vi "Create Evaluations.vi"(8 "error in (no error)":errorcluster, 11 "SPECAN_PVT in":refnum<class "SPECAN_PVT.lvclass">) -> (0 "error out":errorcluster, 1 "Evaluations Out":T1[](array[typedef]) {"Low Limit" format="%#_13g"; "SI Scaling" items=["femto"=-15, "pico"=-12, "nano"=-9, "micro"=-6, "milli"=-3, "percent"=-2, ""=0, "kilo"=3, "mega"=6, "giga"=9, "tera"=12]}, 3 "SPECAN_PVT out":refnum<class "SPECAN_PVT.lvclass">)   [LabVIEW 2018, in "SPECAN_PVT.lvlib" / "SPECAN_PVT.lvclass"]
uses:
  SPECAN_PVT.lvclass
  Plugins/TestStand API Tools (TSAT).lvlibp/Evaluation Actions/Includes/Controls/TSAT Evaluation.ctl
  Plugins/TestStand API Tools (TSAT).lvlibp/Evaluation Actions/Includes/Controls/TSAT Eval SI Unit Scaling.ctl
  Plugins/TestStand API Tools (TSAT).lvlibp/Evaluation Actions/Includes/Controls/TSAT Evaluation Type.ctl
  SPECAN_PVT.lvclass/SPECAN_PVT.ctl
  Plugins/SeqAuto Evaluations.lvlibp/ModeSwitch/ModeSwitch Eval.lvclass
  Plugins/TestStand API Tools (TSAT).lvlibp/Evaluation Actions/TSAT Evaluation Actions.lvlib
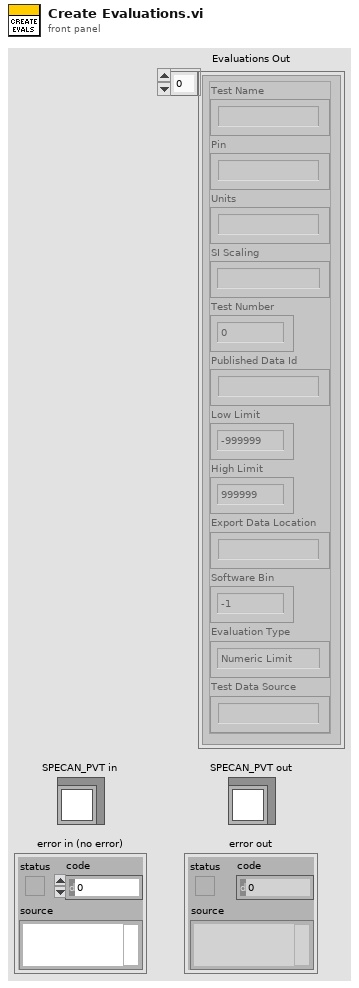
[diagram p1: front panel]
types:
  T1 = typedef "TestStand API Tools (TSAT).lvlibp/TSAT Evaluation Actions.lvlib/TSAT Evaluation.ctl" = cluster{"Test Name":string, "Pin":string, "Units":string, "SI Scaling":T2, "Test Number":i32, "Published Data Id":string, "Low Limit":dbl, "High Limit":dbl, "Export Data Location":string, "Software Bin":i64, "Evaluation Type":T3, "Test Data Source":string}
  T2 = typedef "TestStand API Tools (TSAT).lvlibp/TSAT Evaluation Actions.lvlib/TSAT Eval SI Unit Scaling.ctl" = i16
  T3 = typedef "TestStand API Tools (TSAT).lvlibp/TSAT Evaluation Actions.lvlib/TSAT Evaluation Type.ctl" = enum16{"Numeric Limit", "Pass/Fail", "None"}
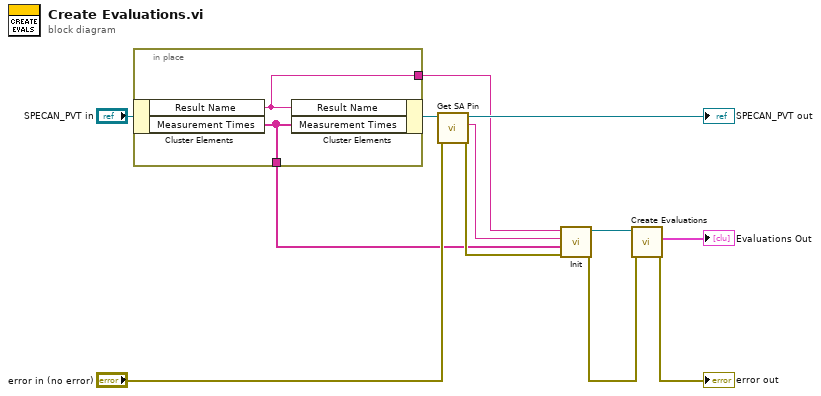
[diagram p0: block diagram]
diagram:
  n1 = in-place {
    in-place-border: [w14] -> w4
    in-place-border: [w13] -> w1
    n2 = in-place-cluster #1("SPECAN_PVT in") -> ("Result Name"=w13:string, "Measurement Times"=w14:string[])
    n3 = in-place-cluster #1("Result Name"=w13, "Measurement Times"=w14) -> (w6:refnum<class "SPECAN_PVT.lvclass">)
  }
  n4 = call-dynamic "Get SA Pin.vi"("error in (no error)"="error in (no error)", "SPECAN_PVT in"=w6) -> ("error out"=w9:errorcluster, "SA PIN"=w8:string, "SPECAN_PVT out"=→"SPECAN_PVT out":refnum<class "SPECAN_PVT.lvclass">)  [unwired: 7 in]
  n5 = call "Init.vi"("error in (no error)"=w9, "Measurement Times"=w4, "SA Pin"=w8, "Measurement Name"=w1) -> ("error out"=w11:errorcluster, "ModeSwitch Eval out"=w12:refnum<class "ModeSwitch Eval.lvclass">)  [unwired: 6 in]
  n6 = call-dynamic "Create Evaluations.vi"("error in (no error)"=w11, "IEvaluation in"=w12) -> ("error out"=→"error out":errorcluster, "Evaluations Out"=→"Evaluations Out":T1[])  [unwired: 7 in, 1 out]
